vi "get trigger.vi"(8 "error in (no error)":errorcluster, 11 "Thorcam in":refnum<class "Thorcam.lvclass">) -> (0 "error out":errorcluster, 3 "Thorcam out":refnum<class "Thorcam.lvclass">)   [LabVIEW 2012, in "Thorcam.lvclass"]
uses:
  Thorcam.lvclass
  Thorcam.lvclass/Thorcam.ctl
panel:
  out "Status":i32
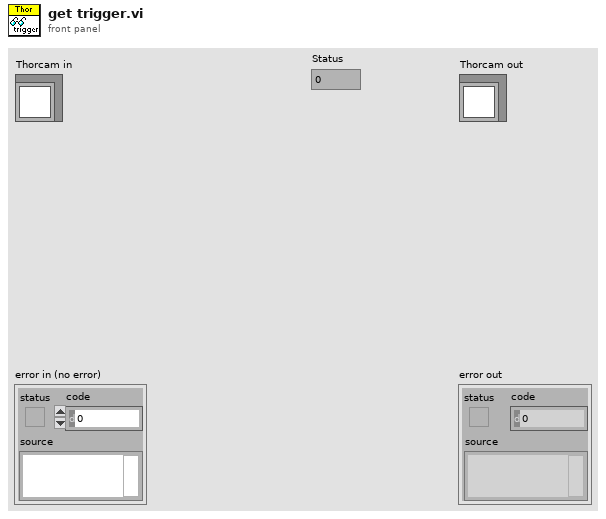
[diagram p1: front panel]
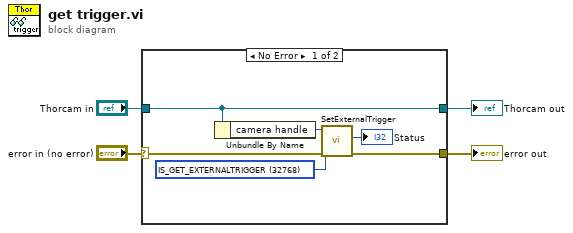
[diagram p0: block diagram]
diagram:
  n1 = case shown="No Error" "error in (no error)" {
    selector: "error in (no error)" -> [w7 w11]
    tunnel: [w7 w11] -> w3
    tunnel: [w9 w10] -> w1
    tunnel: "Thorcam in" -> [w9 w10]
    frame No Error {
      w6 = 32768 items=["IS_SET_TRIG_OFF"=0, "IS_SET_TRIG_HI_LO"=1, "IS_SET_TRIG_LO_HI"=2, "IS_SET_TRIG_SOFTWARE"=8, "IS_GET_EXTERNALTRIGGER"=32768, "IS_GET_TRIGGER_STATUS"=32769] ("Trigger Mode")
      n2 = Unbundle By Name(w9) -> ("camera handle"=w8:u32)
      n3 = call <instrlib>:"SetExternalTrigger.vi"("error in"=w7, "Trigger Mode"=w6, "Camera Handle In"=w8) -> ("Status"=→"Status":i32)  [unwired: 6 in, 2 out]
    }
    frame Error {
    }
  }
  "error out" <- w3
  "Thorcam out" <- w1
